vi "auto_Trans.vi"() -> ()   [LabVIEW 2016]
uses:
  <vilib>/Utility/miscctls.llb/LVOffsetAndMultiplierTypeDef.ctl
panel:
  in  "Tab Control":enum32{"Settings", "Raw", "Intensity"}(tab)
  out "Index":T1={"B Field"=1, "Voltage 2"=6, "Voltage 1"=4, "Current"=10, "Side Gate"=3, "Single/Differential 2"=FALSE} {"Side Gate" items=["time", "Vsg", "T", "B", "X0", "Y0", "X1", "Y1", "X2", "Y2", "X3", "Y3", "X4", "Y4", "X5", "Y5", "B_rate", "R4t(e2/h)", "axis1", "axis2", "20", "21", "22", "23", "24", "25", "26", "27", ""]; "Current" items=["time", "Vsg", "T", "B", "X0", "Y0", "X1", "Y1", "X2", "Y2", "X3", "Y3", "X4", "Y4", "X5", "Y5", "B_rate", "R4t(e2/h)", "axis1", "axis2", "20", "21", "22", "23", "24", "25", "26", "27", ""]; "Voltage 1" items=["time", "Vsg", "T", "B", "X0", "Y0", "X1", "Y1", "X2", "Y2", "X3", "Y3", "X4", "Y4", "X5", "Y5", "B_rate", "R4t(e2/h)", "axis1", "axis2", "20", "21", "22", "23", "24", "25", "26", "27", ""]; "Voltage 2" items=["time", "Vsg", "T", "B", "X0", "Y0", "X1", "Y1", "X2", "Y2", "X3", "Y3", "X4", "Y4", "X5", "Y5", "B_rate", "R4t(e2/h)", "axis1", "axis2", "20", "21", "22", "23", "24", "25", "26", "27", ""]; "B Field" items=["time", "Vsg", "T", "B", "X0", "Y0", "X1", "Y1", "X2", "Y2", "X3", "Y3", "X4", "Y4", "X5", "Y5", "B_rate", "R4t(e2/h)", "axis1", "axis2", "20", "21", "22", "23", "24", "25", "26", "27", ""]}
  in  "Derivative Bin \nSize":dbl=20.0
  out "Comments":string="IGOR\nX// Date: 1/22/2017 12:53 AM\nX// sweep B: 0T to 18T and 18T to 0T, @ 0.02 T/min\nX// sweep Vsg: 0mV to 120mV, 250uV steps\nX// Vbg=0.3V\nX// T~20mK\nX// \nX// lockin settings: \nX// tc=0.3s\nX// order=4\nX// prefilters OFF\nX// \nX// 0: 1, voltage\nX// 1: 2, current, 100uV AC 240uV DC, 13 Hz\nX// 2: 3, voltage\nX// 3: 4, voltage\nX// 4: 5, current\nX// 5: 7, voltage\nX//  \nX// KH gian=100x, shurt resistor=50kOhm\nX// \nX// angle=167.007000\n\n\n\n\n\n\n\n\n\n\n\n\n\n\n\n\n\n\n\n\n\n\n\n\n\n\n\n\n\n\n\n\n\n\n\n\n\n\n\n\n\n\nX \nX Display/R 'time.SA02836H.20170110.000534'\nX AppendToGraph 'Vsg.SA02836H.20170110.000534'\nX AppendToGraph 'T.SA02836H.20170110.000534'\nX AppendToGraph 'B.SA02836H.20170110.000534'\nX AppendToGraph 'X0.SA02836H.20170110.000534'\nX AppendToGraph 'Y0.SA02836H.20170110.000534'\nX AppendToGraph 'X1.SA02836H.20170110.000534'\nX AppendToGraph 'Y1.SA02836H.20170110.000534'\nX AppendToGraph 'X2.SA02836H.20170110.000534'\nX AppendToGraph 'Y2.SA02836H.20170110.000534'\nX AppendToGraph 'X3.SA02836H.20170110.000534'\nX AppendToGraph 'Y3.SA02836H.20170110.000534'\nX AppendToGraph 'X4.SA02836H.20170110.000534'\nX AppendToGraph 'Y4.SA02836H.20170110.000534'\nX AppendToGraph 'X5.SA02836H.20170110.000534'\nX AppendToGraph 'Y5.SA02836H.20170110.000534'\nX AppendToGraph 'B_rate.SA02836H.20170110.000534'\nX AppendToGraph 'R4t(e2/h).SA02836H.20170110.000534'\nX AppendToGraph 'axis1.SA02836H.20170110.000534'\nX AppendToGraph 'axis2.SA02836H.20170110.000534'\nX Label bottom \"x label\"\nX Label left \"y label\"\nX ModifyGraph rgb('time.SA02836H.20170110.000534')=(65280,0,0)\nX ModifyGraph rgb('Vsg.SA02836H.20170110.000534')=(65280,18432,0)\nX ModifyGraph rgb('T.SA02836H.20170110.000534')=(65280,35328,0)\nX ModifyGraph rgb('B.SA02836H.20170110.000534')=(65280,52224,0)\nX ModifyGraph rgb('X0.SA02836H.20170110.000534')=(60416,65280,0)\nX ModifyGraph rgb('Y0.SA02836H.20170110.000534')=(41984,65280,0)\nX ModifyGraph rgb('X1.SA02836H.20170110.000534')=(25088,65280,0)\nX ModifyGraph rgb('Y1.SA02836H.20170110.000534')=(8192,65280,0)\nX ModifyGraph rgb('X2.SA02836H.20170110.000534')=(0,65280,10240)\nX ModifyGraph rgb('Y2.SA02836H.20170110.000534')=(0,65280,28672)\nX ModifyGraph rgb('X3.SA02836H.20170110.000534')=(0,65280,45568)\nX ModifyGraph rgb('Y3.SA02836H.20170110.000534')=(0,65280,62464)\nX ModifyGraph rgb('X4.SA02836H.20170110.000534')=(0,50176,65280)\nX ModifyGraph rgb('Y4.SA02836H.20170110.000534')=(0,31744,65280)\nX ModifyGraph rgb('X5.SA02836H.20170110.000534')=(0,14848,65280)\nX ModifyGraph rgb('Y5.SA02836H.20170110.000534')=(2048,0,65280)\nX ModifyGraph rgb('B_rate.SA02836H.20170110.000534')=(20480,0,65280)\nX ModifyGraph rgb('R4t(e2/h).SA02836H.20170110.000534')=(38912,0,65280)\nX ModifyGraph rgb('axis1.SA02836H.20170110.000534')=(55808,0,65280)\nX ModifyGraph rgb('axis2.SA02836H.20170110.000534')=(65280,0,58368)\nX Legend/C/N=text0/J \"\\\\s('time.SA02836H.20170110.000534') time\\r\\\\s('Vsg.SA02836H.20170110.000534') Vsg\\r\\\\s('T.SA02836H.20170110.000534') T\\r\\\\s('B.SA02836H.20170110.000534') B\\r\\\\s('X0.SA02836H.20170110.000534') X0\\r\\\\s('Y0.SA02836H.20170110.000534') Y0\\r\\\\s('X1.SA02836H.20170110.000534') X1\\r\\\\s('Y1.SA02836H.20170110.000534') Y1\\r\\\\s('X2.SA02836H.20170110.000534') X2\\r\\\\s('Y2.SA02836H.20170110.000534') Y2\\r\\\\s('X3.SA02836H.20170110.000534') X3\\r\\\\s('Y3.SA02836H.20170110.000534') Y3\\r\\\\s('X4.SA02836H.20170110.000534') X4\\r\\\\s('Y4.SA02836H.20170110.000534') Y4\\r\\\\s('X5.SA02836H.20170110.000534') X5\\r\\\\s('Y5.SA02836H.20170110.000534') Y5\\r\\\\s('B_rate.SA02836H.20170110.000534') B_rate\\r\\\\s('R4t(e2/h).SA02836H.20170110.000534') R4t (e2/h)\\r\\\\s('axis1.SA02836H.20170110.000534') axis 1\\r\\\\s('axis2.SA02836H.20170110.000534') axis 2\"\nX ModifyGraph mirror(bottom)=1\nX ModifyGraph width=216\nX ModifyGraph height={Aspect,0.6}\nX ModifyGraph Log(bottom)=0\nX ModifyGraph Log(left)=0\nX \n"
  in  "Index":bool
  in  "Path":path=path "C:/LevyLab/LevyLab Projects/automation/files"
  in  "Index.":T2={"Side Gate"=1, "Current"=12, "Voltage 1"=8, "Voltage 2"=10, "B Field"=3, "Single/Differential 2"=TRUE}
  in  "Stop":bool
  out "Transconductance":T3(graph)
  out "Conductance":T3(graph)
  out "String 2":string="Transconductance"
  out "String":string="Conductance"
  out "Transconductance..":dbl[][](graph)
  out "String 4":string="Transconductance"
  out "Conductance..":dbl[][](graph)
  out "String 3":string="Conductance"
  out "Added?":string="Handle Closed"
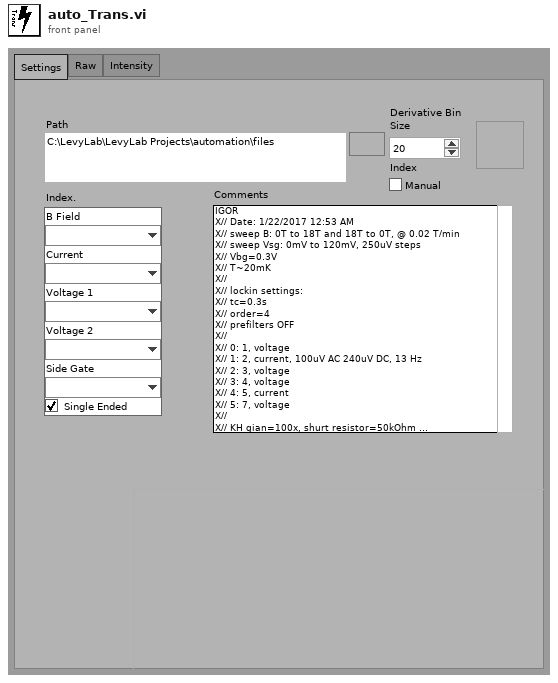
[diagram p1: front panel]
types:
  T1 = cluster{"B Field":i32, "Voltage 2":i32, "Voltage 1":i32, "Current":i32, "Side Gate":i32, "Single/Differential 2":bool}
  T2 = cluster{"Side Gate":i32, "Current":i32, "Voltage 1":i32, "Voltage 2":i32, "B Field":i32, "Single/Differential 2":bool}
  T3 = cluster{"Vfast":dbl[], "Decimated Array":dbl[]}[]
  T4 = enum32{"invalid app kind", "Development System", "Run Time System", "Student Edition", "Embedded LabVIEW", "Evaluation", "Custom"}
  T5 = enum32{"Invalid", "Standard", "Closed", "Hidden", "Minimized", "Maximized"}
  T6 = typedef "LVOffsetAndMultiplierTypeDef.ctl" = cluster{"Offset":dbl, "Multiplier":dbl}
  T7 = cluster{"N1":i32, "N2":i32, "N3":i32, "N4":i32, "V1":i32, "V2":i32, "V3":i32, "V4":i32, "CURRENT":i32, "Vsg":i32}
  T8 = cluster{"Core":cluster{"Current VI Reference":refnum<vi>, "Close Panel on Exit?":bool}, "Boolean Values":cluster{"Your Boolean data":bool, "single ended?":bool}, "Your string data":string, "Paths":cluster{"Path":path}, "Graphs":cluster{"Cond.":cluster{dbl[], dbl[]}[], "Trans.":cluster{"Vfast":dbl[], "Decimated Array":dbl[]}[], "Cond. Intens.":dbl[][], "Trans. Intens.":dbl[][], "Cond. Intens. bg":dbl[][], "Trans. Intens. bg":dbl[][]}, "Index/ Comments":cluster{"Comments":string, "Index":cluster{"N1":i32, "N2":i32, "N3":i32, "N4":i32, "V1":i32, "V2":i32, "V3":i32, "V4":i32, "CURRENT":i32, "Vsg":i32}, "Wavenames":string[]}, "Images":cluster{"Image":picture}, "B Field":i32}
  T9 = cluster{"Comments":string, "Index":cluster{"N1":i32, "N2":i32, "N3":i32, "N4":i32, "V1":i32, "V2":i32, "V3":i32, "V4":i32, "CURRENT":i32, "Vsg":i32}, "Wavenames":string[]}
  T10 = cluster{"Your Boolean data":bool, "single ended?":bool}
  T11 = cluster{"Cond.":cluster{dbl[], dbl[]}[], "Trans.":cluster{"Vfast":dbl[], "Decimated Array":dbl[]}[], "Cond. Intens.":dbl[][], "Trans. Intens.":dbl[][], "Cond. Intens. bg":dbl[][], "Trans. Intens. bg":dbl[][]}
  T12 = cluster{"Current VI Reference":refnum<vi>, "Close Panel on Exit?":bool}
  T13 = cluster{"Side Gate":i32, "Current":i32, "Voltage 1":i32, "Voltage 2":i32, "B Field":i32, "Voltage":bool}
  T14 = cluster{"Decimated Array":dbl[], "Decimated Array":dbl[]}
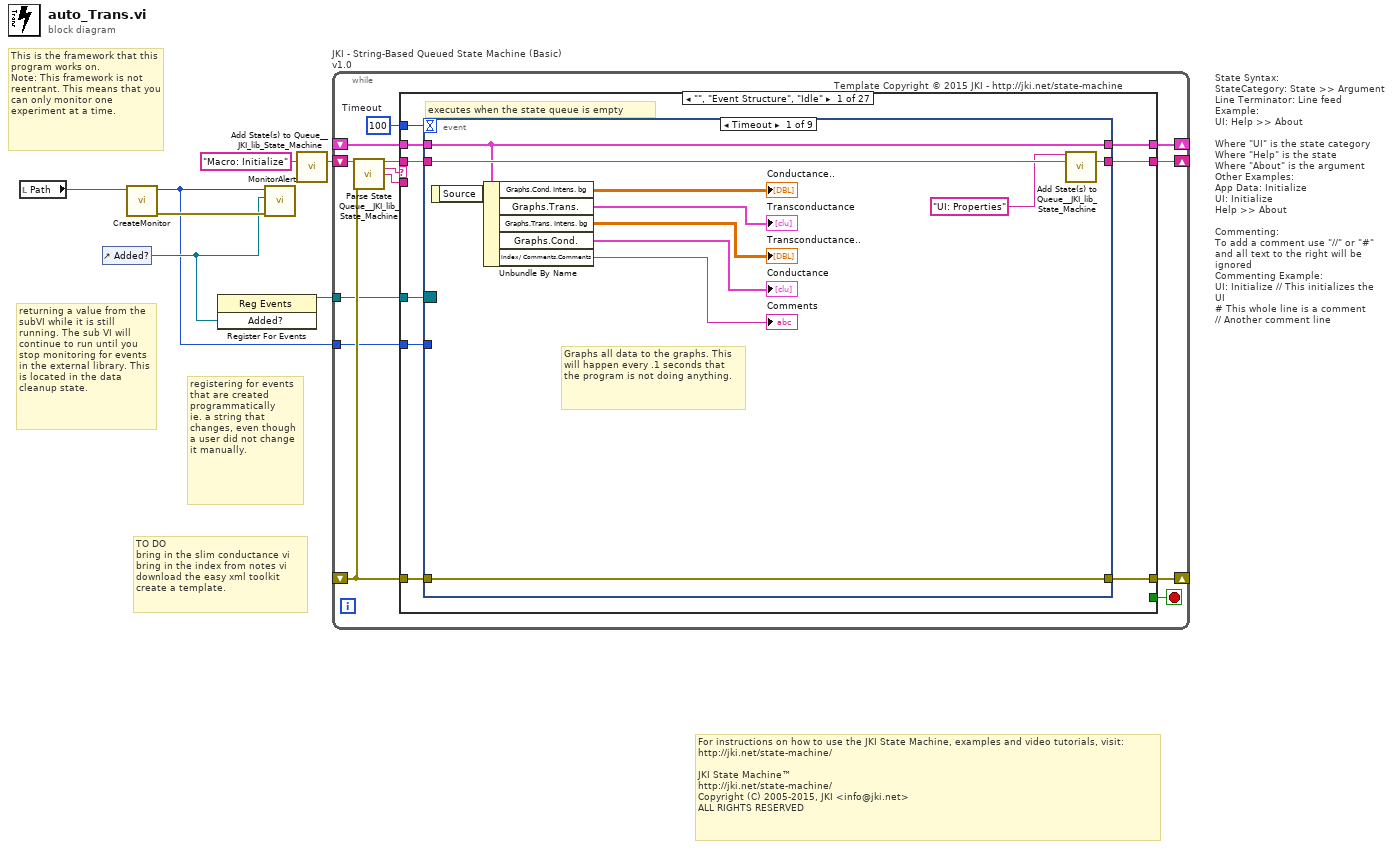
[diagram p0: block diagram]
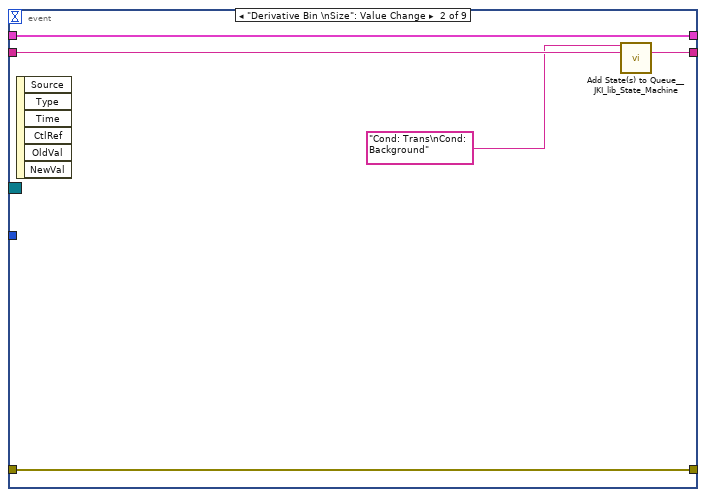
[diagram p2: hidden frame]
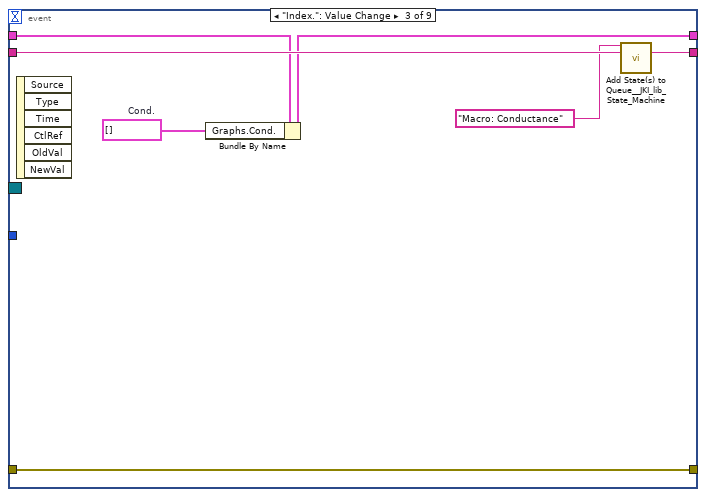
[diagram p3: hidden frame]
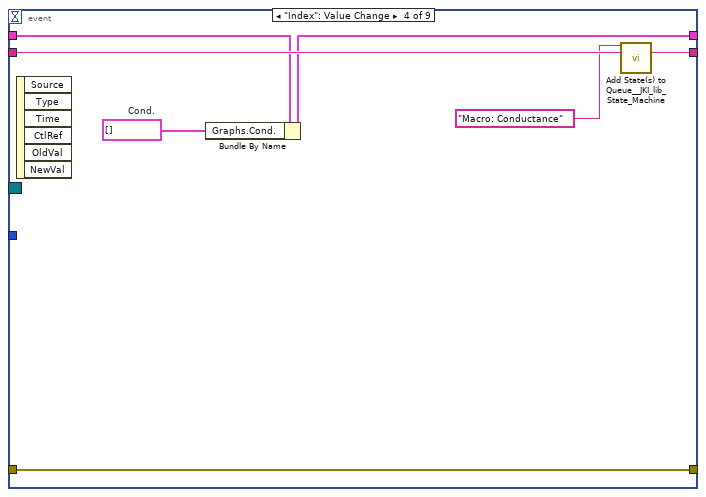
[diagram p4: hidden frame]
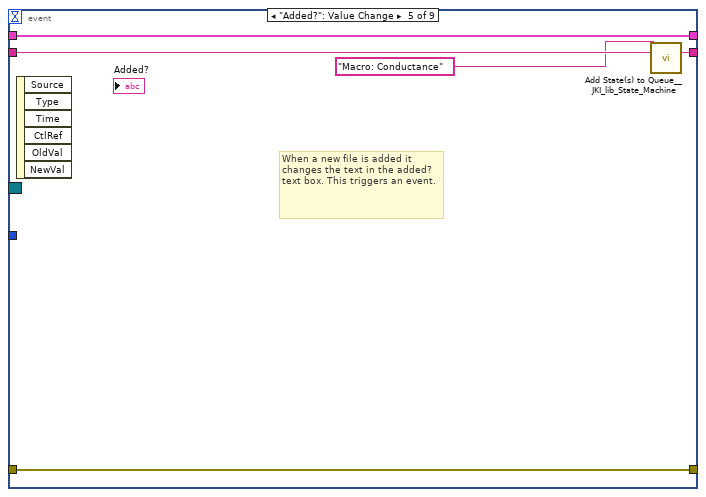
[diagram p5: hidden frame]
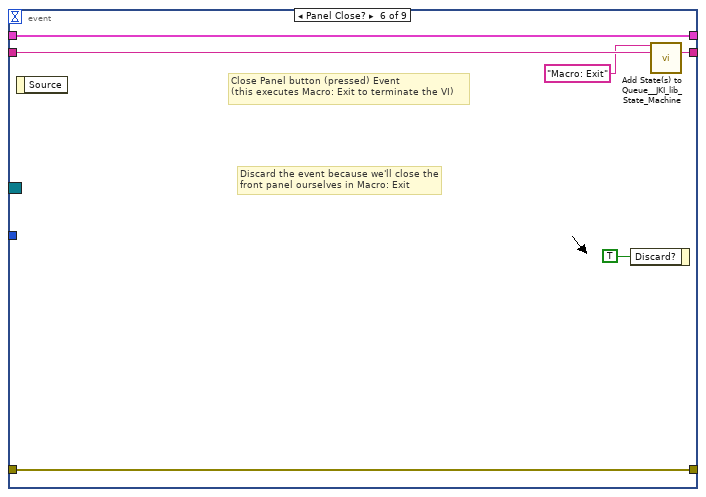
[diagram p6: hidden frame]
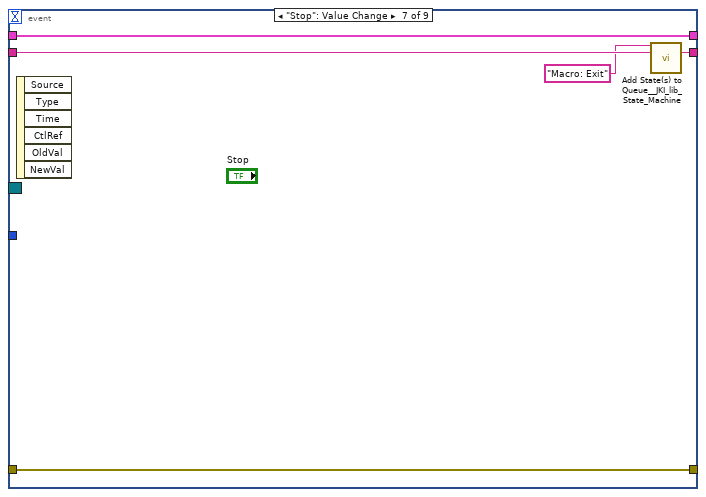
[diagram p7: hidden frame]
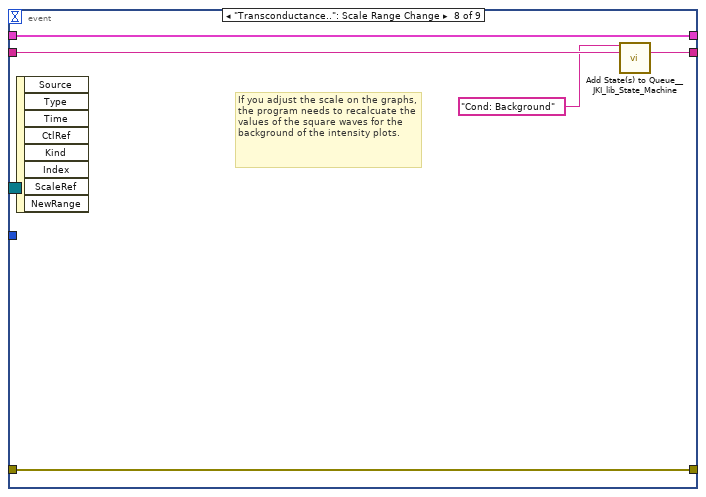
[diagram p8: hidden frame]
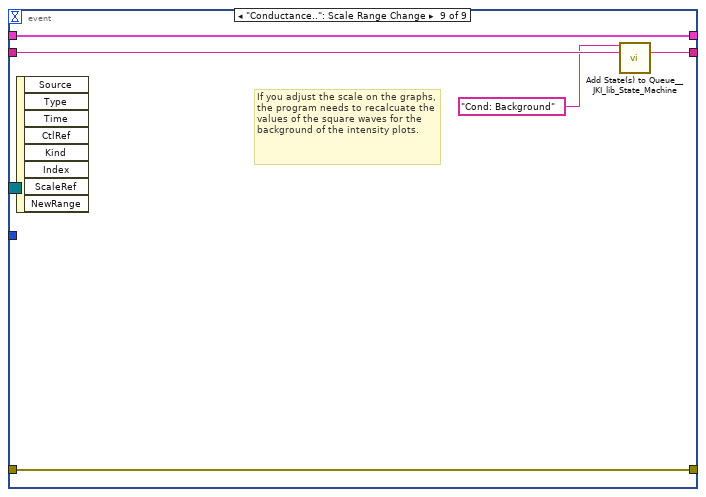
[diagram p9: hidden frame]
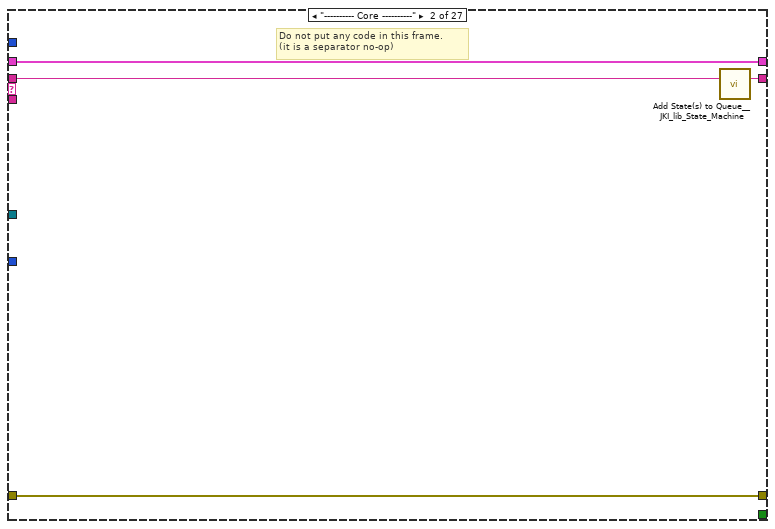
[diagram p10: hidden frame]
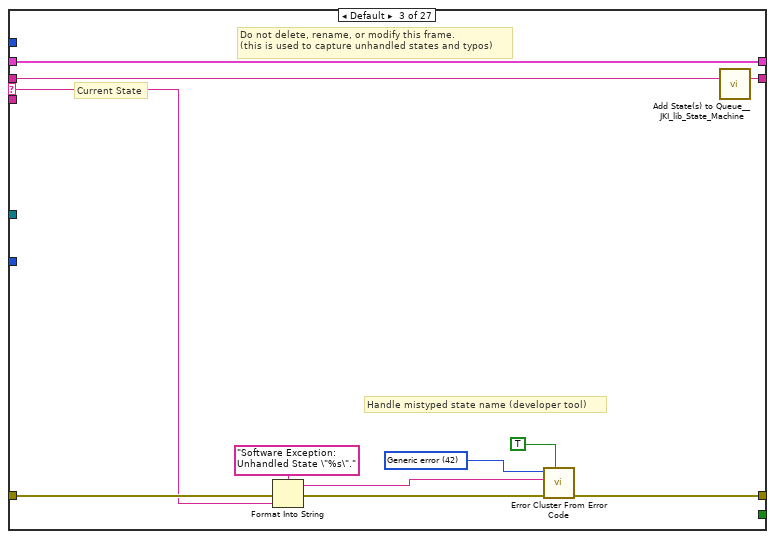
[diagram p11: hidden frame]
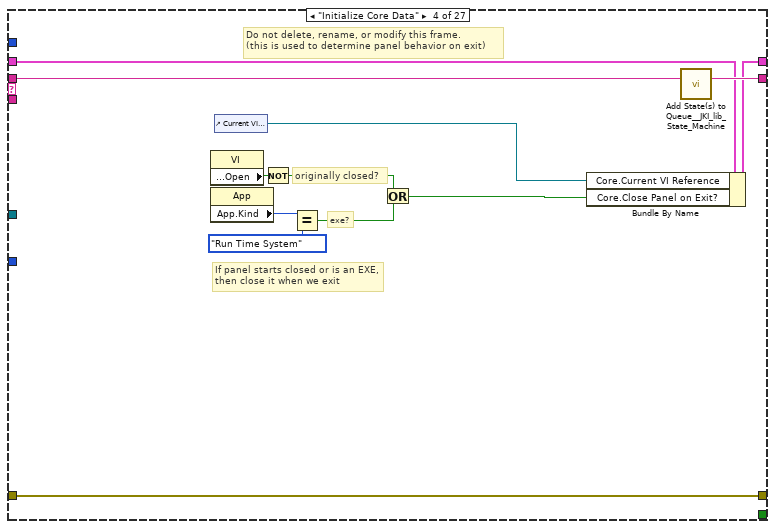
[diagram p12: hidden frame]
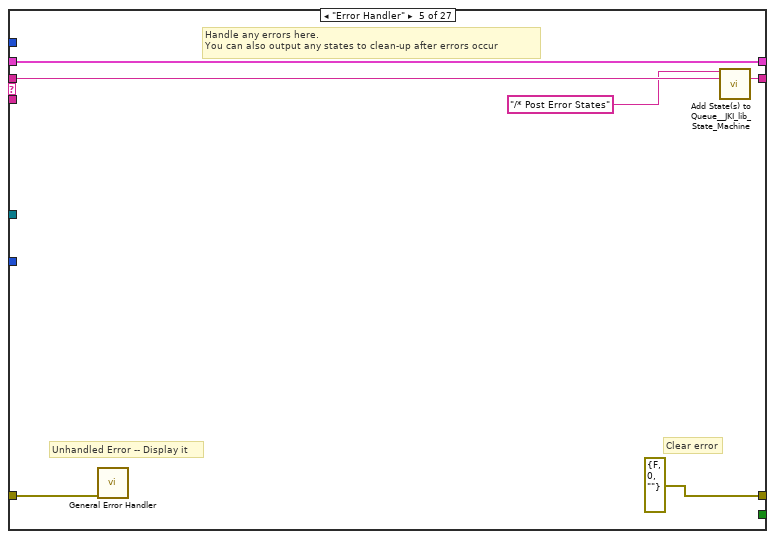
[diagram p13: hidden frame]
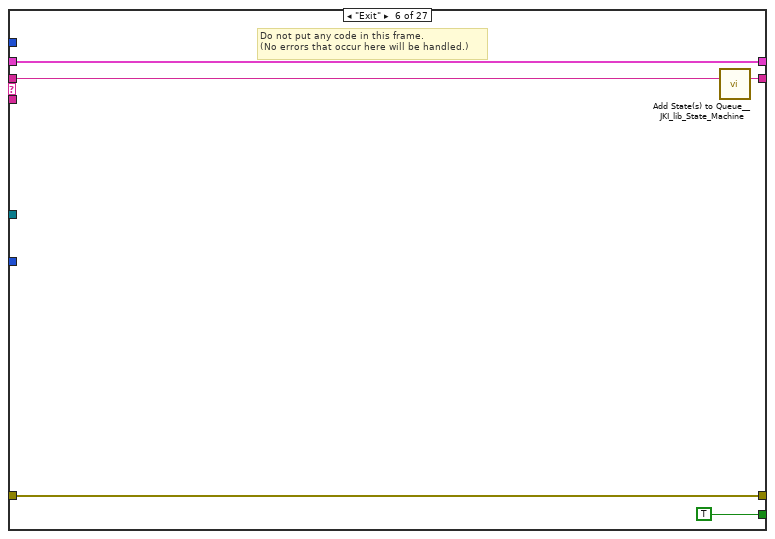
[diagram p14: hidden frame]
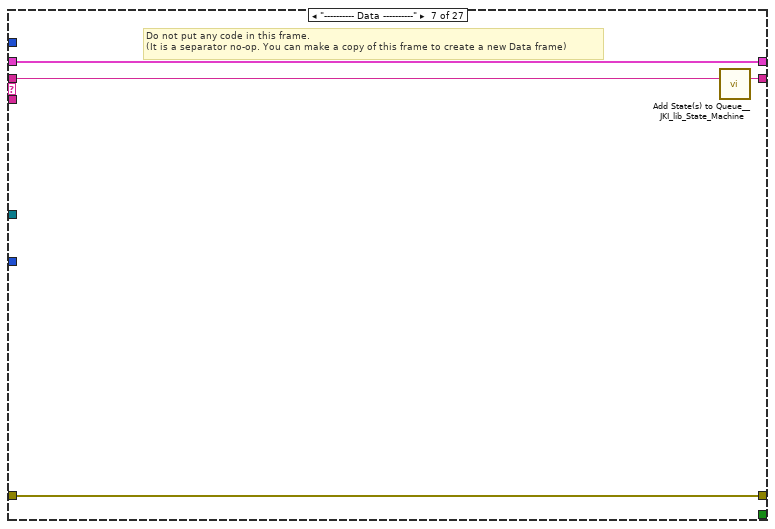
[diagram p15: hidden frame]
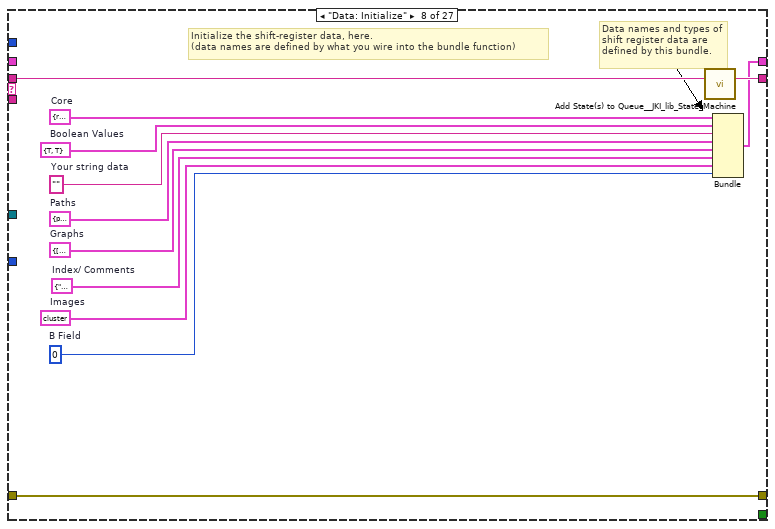
[diagram p16: hidden frame]
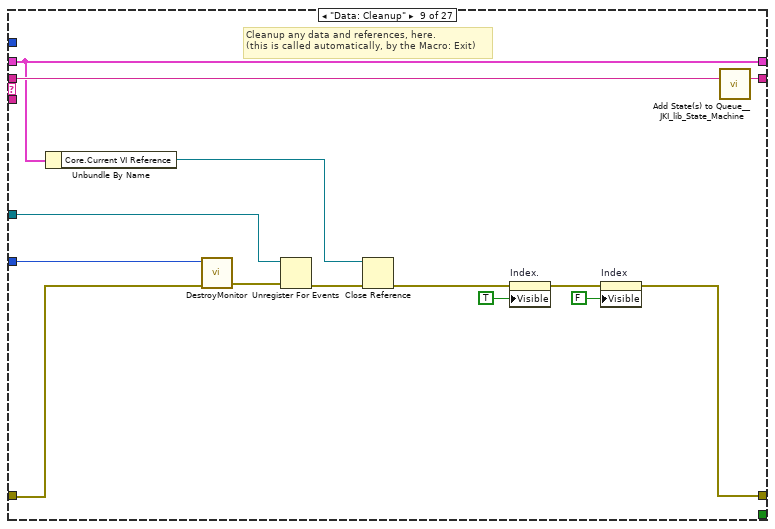
[diagram p17: hidden frame]
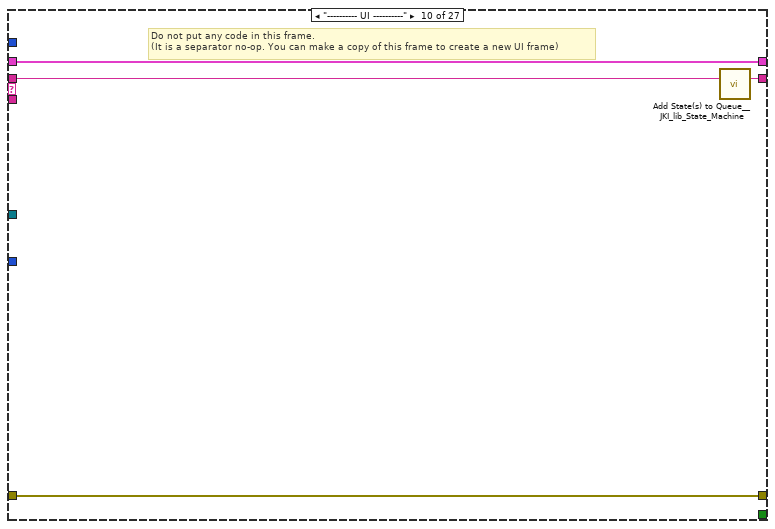
[diagram p18: hidden frame]
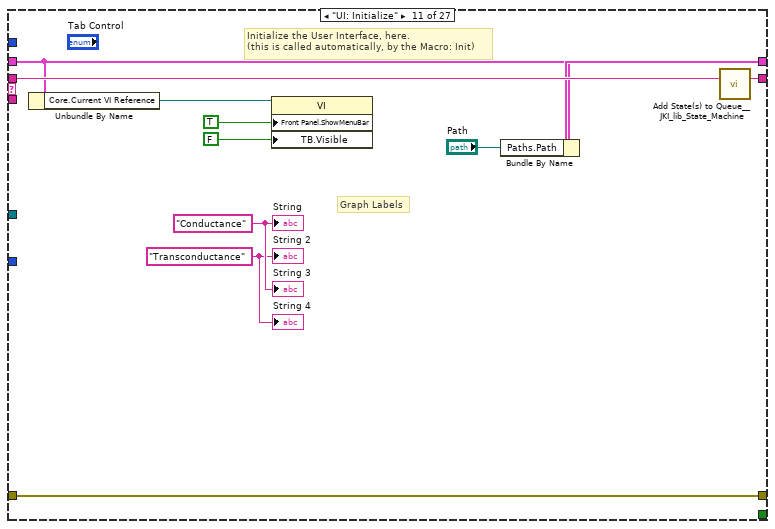
[diagram p19: hidden frame]
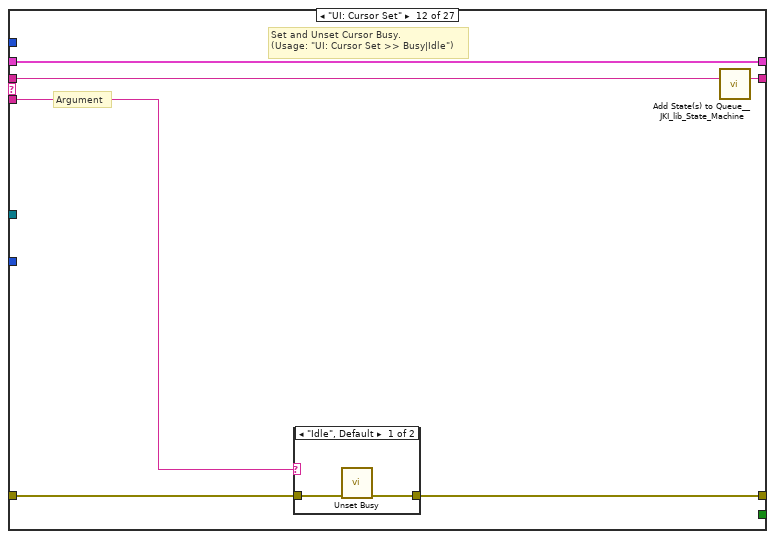
[diagram p20: hidden frame]
diagram:
  # "TO DO\nbring in the slim conductance vi\nbring in the index from notes vi\ndownload the easy xml toolkit\ncreate a template."
  # "registering for events that are created programmatically\nie. a string that changes, even though a user did not change it manually."
  # "returning a value from the subVI while it is still running. The sub VI will continue to run until you stop monitoring for events in the external library. This is located in the data cleanup state."
  # "This is the framework that this program works on.\nNote: This framework is not reentrant. This means that you can only monitor one experiment at a time."
  # "State Syntax:\nStateCategory: State >> Argument\nLine Terminator: Line feed\nExample:\nUI: Help >> About\n\nWhere \"UI\" is the state category\nWhere \"Help\" is the state\nWhere \"About\" is the argument\nOther Examples:\nApp Data: Initialize\nUI: Initialize\nHelp >> About\n\nCommenting:\nTo add a comment use \"//\" or \"#\" and all text to the right will be ignored\nCommenting Example:\nUI: Initialize // This initializes the UI\n# This whole line is a comment\n// Another comment line"
  # "For instructions on how to use the JKI State Machine, examples and video tutorials, visit:\nhttp://jki.net/state-machine/\n\nJKI State Machine™\nhttp://jki.net/state-machine/\nCopyright (C) 2005-2015, JKI <info@jki.net>\nALL RIGHTS RESERVED"
  n1 = local read "Path"() -> (w1:path)
  n2 = control-ref of="Added?"() -> (w4:refnum<vi>)
  n3 = call "CreateMonitor.vi"("File Path Control"=w1) -> ("error out"=w5:errorcluster, "Handle"=w2:i32)  [unwired: 9 in]
  n4 = register-events(w4) -> (reference out=w3:refnum<event-registration>)  [unwired: 2 in, 1 out]
  n5 = call "MonitorAlert.vi"("error in (no error)"=w5, "Str Refnum"=w4, "Handle"=w2) -> ()  [unwired: 8 in, 1 out]
  n6 = call <vilib>:"Add State(s) to Queue__JKI_lib_State_Machine.vi"("State(s) in (\"\")"="Macro: Initialize") -> ("States Out"=w7:string)  [unwired: 14 in]
  n7 = while "JKI - String-Based Queued State Machine (Basic) v1.0" {
    shift-right: [w13] -> _
    shift-left: _ -> [w12]
    shift-right: [w16] -> _
    shift-left: _ -> [w10]
    shift-right: [w15] -> _
    shift-left: w7 -> [w17]
    tunnel: w3 -> [w9]
    tunnel: w2 -> [w8]
    stop <- w14 stop-if-true
    w11 = 100  # Timeout
    # "Template Copyright © 2015 JKI - http://jki.net/state-machine"
    n8 = call <vilib>:"Parse State Queue__JKI_lib_State_Machine.vi"("State Queue"=w17, "Error In (no error)"=w10) -> ("Remaining States"=w19:string, "Current State"=w20:string, "Arguments"=w18:string)  [unwired: 11 in]
    n9 = case shown="\"\", \"Event Structure\", \"Idle\"" w20 {
      selector: w20 -> [_ _ w89 _ _ _ _ _ _ _ _ _ _ _ _ _ _ _ _ _ _ _ _ _ _ _ _]
      tunnel: w19 -> [w29 w88 w93 w111 w117 w122 w126 w138 w152 w156 w167 w173 w184 w228 w234 w239 w244 w254 w258 w269 w273 w294 w315 w325 w343 w347 w351]
      tunnel: w18 -> [_ _ _ _ _ _ _ _ _ _ _ w168 w178 _ _ _ _ _ _ _ _ _ _ _ _ _ _]
      tunnel: w12 -> [w27 w85 w91 w102 w114 w120 w123 _ w150 w153 w163 w171 w180 w225 w231 w236 w241 w252 w255 w267 w270 w287 w311 w318 w340 w344 w348]
      tunnel: [w26 w86 w95 w108 errorcluster {"status"=FALSE, "code"=0, "source"=""} ("error out") w119 w124 w135 w140 w154 w164 w169 w181 w226 w232 w237 w242 w245 w256 w259 w271 w292 w313 w323 w341 w345 w349] -> w16
      tunnel: w10 -> [w25 w86 w94 w108 w113 w119 w124 w135 w144 w154 w164 w170 w182 w226 w232 w237 w242 w245 w256 w260 w271 w292 w313 w323 w341 w345 w349]
      tunnel: [w28 w87 w92 w110 w116 w121 w125 w137 w151 w155 w166 w172 w183 w227 w233 w238 w243 w253 w257 w268 w272 w293 w314 w324 w342 w346 w350] -> w15
      tunnel: [_ _ _ _ _ TRUE _ _ _ _ _ _ _ _ _ _ _ _ _ _ _ _ _ _ _ _ _] -> w14
      tunnel: [w24 w85 w91 w109 w114 w120 w123 w136 w150 w153 w165 w171 w180 w225 w231 w236 w241 w252 w255 w267 w270 w286 w312 w320 w339 w344 w348] -> w13
      tunnel: w11 -> [w23 _ _ _ _ _ _ _ _ _ _ _ _ _ _ _ _ _ _ _ _ _ _ _ _ _ _]
      tunnel: w9 -> [w22 _ _ _ _ _ _ _ w148 _ _ _ _ _ _ _ _ _ _ _ _ _ _ _ _ _ _]
      tunnel: w8 -> [w21 _ _ _ _ _ _ _ w149 _ _ _ _ _ _ _ _ _ _ _ _ _ _ _ _ _ _]
      frame "", "Event Structure", "Idle" {
        # "executes when the state queue is empty"
        n10 = event shown="[0] Timeout" {
          selector: w22 -> [_ _ _ _ _ _ _ _ _]
          dyn-events: _ -> [_ _ _ _ _ _ _ _ _]
          timeout: w23 -> [_ _ _ _ _ _ _ _ _]
          tunnel: w29 -> [w39 w42 w49 w56 w63 w69 w74 w77 w82]
          tunnel: [w38 w43 w50 w57 w62 w68 w73 w78 w83] -> w28
          tunnel: w27 -> [w36 w41 w46 w53 w61 w66 w71 w79 w84]
          tunnel: [w37 w44 w51 w58 w60 w67 w72 w75 w80] -> w26
          tunnel: w25 -> [w37 w44 w51 w58 w60 w67 w72 w75 w80]
          tunnel: [w36 w41 w45 w52 w61 w66 w71 w79 w84] -> w24
          tunnel: w21 -> [_ _ _ _ _ _ _ _ _]
          event Timeout {
            # "Graphs all data to the graphs. This will happen every .1 seconds that the program is not doing anything."
            n11 = event-data() -> ()  [unwired: 1 in, 1 out]
            n12 = Unbundle By Name(w36) -> ("Graphs.Cond. Intens. bg"=→"Conductance..":dbl[][], "Graphs.Trans."=→"Transconductance":T3, "Graphs.Trans. Intens. bg"=→"Transconductance..":dbl[][], "Graphs.Cond."=→"Conductance":cluster{dbl[], dbl[]}[], "Index/ Comments.Comments"=→"Comments":string)
            n13 = call <vilib>:"Add State(s) to Queue__JKI_lib_State_Machine.vi"("State(s) in Front (\"\")"="UI: Properties" ("State(s) in Front (\"\")"), "State(s) in (\"\")"=w39) -> ("States Out"=w38:string)  [unwired: 13 in]
          }
          event "Derivative Bin \nSize": Value Change {
            n14 = event-data() -> ()  [unwired: 1 in, 6 out]
            n15 = call <vilib>:"Add State(s) to Queue__JKI_lib_State_Machine.vi"("State(s) in Front (\"\")"="Cond: Trans\nCond: Background" ("State(s) in Front (\"\")"), "State(s) in (\"\")"=w42) -> ("States Out"=w43:string)  [unwired: 13 in]
          }
          event "Index.": Value Change {
            w48 = cluster{dbl[], dbl[]}[] []  # Cond.
            n16 = event-data() -> ()  [unwired: 1 in, 6 out]
            n17 = Bundle By Name(cluster=w46, "Graphs.Cond."=w48) -> (w45:T8)
            n18 = call <vilib>:"Add State(s) to Queue__JKI_lib_State_Machine.vi"("State(s) in Front (\"\")"="Macro: Conductance" ("State(s) in Front (\"\")"), "State(s) in (\"\")"=w49) -> ("States Out"=w50:string)  [unwired: 13 in]
          }
          event "Index": Value Change {
            w55 = cluster{dbl[], dbl[]}[] []  # Cond.
            n19 = event-data() -> ()  [unwired: 1 in, 6 out]
            n20 = Bundle By Name(cluster=w53, "Graphs.Cond."=w55) -> (w52:T8)
            n21 = call <vilib>:"Add State(s) to Queue__JKI_lib_State_Machine.vi"("State(s) in Front (\"\")"="Macro: Conductance" ("State(s) in Front (\"\")"), "State(s) in (\"\")"=w56) -> ("States Out"=w57:string)  [unwired: 13 in]
          }
          event "Added?": Value Change {
            # "When a new file is added it changes the text in the added? text box. This triggers an event."
            n22 = event-data() -> ()  [unwired: 1 in, 6 out]
            n23 = call <vilib>:"Add State(s) to Queue__JKI_lib_State_Machine.vi"("State(s) in Front (\"\")"="Macro: Conductance" ("State(s) in Front (\"\")"), "State(s) in (\"\")"=w63) -> ("States Out"=w62:string)  [unwired: 13 in]
          }
          event Panel Close? {
            # "Discard the event because we'll close the front panel ourselves in Macro: Exit"
            # "Close Panel button (pressed) Event\n(this executes Macro: Exit to terminate the VI)"
            n24 = event-data() -> ()  [unwired: 1 in, 1 out]
            n25 = event-data("Discard?"=TRUE) -> ()  [unwired: 1 in, 1 out]
            n26 = call <vilib>:"Add State(s) to Queue__JKI_lib_State_Machine.vi"("State(s) in Front (\"\")"="Macro: Exit", "State(s) in (\"\")"=w69) -> ("States Out"=w68:string)  [unwired: 13 in]
          }
          event "Stop": Value Change {
            n27 = event-data() -> ()  [unwired: 1 in, 6 out]
            n28 = call <vilib>:"Add State(s) to Queue__JKI_lib_State_Machine.vi"("State(s) in Front (\"\")"="Macro: Exit", "State(s) in (\"\")"=w74) -> ("States Out"=w73:string)  [unwired: 13 in]
          }
          event "Transconductance..": Scale Range Change {
            # "If you adjust the scale on the graphs, the program needs to recalcuate the values of the square waves for the background of the intensity plots."
            n29 = event-data() -> ()  [unwired: 1 in, 8 out]
            n30 = call <vilib>:"Add State(s) to Queue__JKI_lib_State_Machine.vi"("State(s) in Front (\"\")"="Cond: Background" ("State(s) in Front (\"\")"), "State(s) in (\"\")"=w77) -> ("States Out"=w78:string)  [unwired: 13 in]
          }
          event "Conductance..": Scale Range Change {
            # "If you adjust the scale on the graphs, the program needs to recalcuate the values of the square waves for the background of the intensity plots."
            n31 = event-data() -> ()  [unwired: 1 in, 8 out]
            n32 = call <vilib>:"Add State(s) to Queue__JKI_lib_State_Machine.vi"("State(s) in Front (\"\")"="Cond: Background" ("State(s) in Front (\"\")"), "State(s) in (\"\")"=w82) -> ("States Out"=w83:string)  [unwired: 13 in]
          }
        }
      }
      frame "---------- Core ----------" {
        # "Do not put any code in this frame.\n(it is a separator no-op)"
        n33 = call <vilib>:"Add State(s) to Queue__JKI_lib_State_Machine.vi"("State(s) in (\"\")"=w88) -> ("States Out"=w87:string)  [unwired: 14 in]
      }
      frame Default {
        w98 = 42 items=["No error", "Argument error", "Memory is full", "Out of zone", "End of file", "File already open", "Generic file I/O error", "File not found", "File permission error", "Disk is full", "Duplicate path", "Too many files open", "System feature not enabled", "Resource file not found", "Cannot add resource", "Resource not found", "Image not found", "Image memory error", "Pen does not exist", "Config type invalid", "Config token not found", "Config parse error", "Config memory error", "Bad external code format", "Bad external code offset", "External code not present", "Null window", "Destroy window error", "Null menu", "Print aborted", "Bad print record", "Print driver error", "Windows error during printing", "Memory error during printing", "Print dialog error", "Generic print error", "Invalid device refnum", "Device not found", "Device parameter error", "Device unit error", "Cannot open device", "Device call aborted", "Generic error", "Cancelled by user", "Object ID too low", "Object ID too high", "Object not in heap", "Unknown heap", "Unknown object (invalid DefProc)", "Unknown object (DefProc not in table)", "Message out of range", "Invalid (null) method", "Unknown message", "Manager call not supported", "Bad address", "Network operation in progress", "Network operation timed out", "Connection is busy", "Network attribute not supported", "Network error", "Address in use", "System out of memory", "Connection aborted", "Connection refused", "Not connected", "Already connected", "Connection closed", "Initialization error (interapplication manager)", "Bad occurrence", "Wait on unbound occurrence handler", "Occurrence queue overflow", "Datalog type conflict", "Unused", "Unrecognized type (interapplication manager)", "Memory corrupt", "Failed to make temporary DLL", "Old CIN version", "Drag socket not found", "Failed to load drop-object", "Failed to register OLE object", "Failed to release OLE object", "Format specifier type mismatch", "Unknown format specifier", "Too few format specifiers", "Too many format specifiers", "Scan failed", "Newer CIN version", "Error converting to variant", "Runtime menu error", "Password tampered", "Variant attribute not found", "Incompatible variant data type", "Event data is not available", "Event Store is not present", "Occurrence is not found", "Event Queue is not created", "Event info is not available", "Refnum passed is NULL", "Error retrieving Class GUID", "Error retrieving CoClass GUID", "Error retrieving TypeLib GUID.", "Bad built application magic bytes.", "Specific driver is different from the specific driver associated with the Logical Name.", "There is no session opened to the class driver.", "Max Error", "MAX - Error with config objects", "MAX - Error loading configuration", "MAX - Group not supported"]
        # "Current State"
        # "Do not delete, rename, or modify this frame.\n(this is used to capture unhandled states and typos)"
        # "Handle mistyped state name (developer tool)"
        n34 = Format Into String(format string="Software Exception: Unhandled State \"%s\"." ("message"), error in=w94, w89) -> (resulting string=w97:string, error out=w96:errorcluster)  [unwired: 1 in]
        n35 = call <vilib>:"Error Cluster From Error Code.vi"("show call chain? (False)"=TRUE, "error in (no error)"=w96, "error message (\"\")"=w97, "error code (0)"=w98) -> ("error out"=w95:errorcluster)  [unwired: 5 in]
        n36 = call <vilib>:"Add State(s) to Queue__JKI_lib_State_Machine.vi"("State(s) in (\"\")"=w93) -> ("States Out"=w92:string)  [unwired: 14 in]
      }
      frame "Initialize Core Data" {
        # "Do not delete, rename, or modify this frame.\n(this is used to determine panel behavior on exit)"
        # "originally closed?"
        # "exe?"
        # "If panel starts closed or is an EXE, then close it when we exit"
        n37 = property class="VI"() -> ("Front Panel.Open"=w107:bool)  [unwired: 2 in, 2 out]
        n38 = property class="App"() -> ("App.Kind"=w106:T4)  [unwired: 2 in, 2 out]
        n39 = control-ref of="Current VI Reference"() -> (w100:refnum<vi>)
        n40 = Not(x=w107) -> (.not. x?=w104:bool)
        n41 = Equal?(x=w106, y=T4."Run Time System" ("Application:Kind")) -> (x = y?=w103:bool)
        n42 = Or(x=w104, y=w103) -> (x .or. y?=w101:bool)
        n43 = Bundle By Name(cluster=w102, "Core.Current VI Reference"=w100, "Core.Close Panel on Exit?"=w101) -> (w109:T8)
        n44 = call <vilib>:"Add State(s) to Queue__JKI_lib_State_Machine.vi"("State(s) in (\"\")"=w111) -> ("States Out"=w110:string)  [unwired: 14 in]
      }
      frame "Error Handler" {
        # "Unhandled Error -- Display it"
        # "Handle any errors here.\nYou can also output any states to clean-up after errors occur"
        # "Clear error"
        n45 = call <vilib>:"General Error Handler.vi"("error in (no error)"=w113) -> ()  [unwired: 10 in, 5 out]
        n46 = call <vilib>:"Add State(s) to Queue__JKI_lib_State_Machine.vi"("State(s) in Front (\"\")"="/* Post Error States", "State(s) in (\"\")"=w117) -> ("States Out"=w116:string)  [unwired: 13 in]
      }
      frame "Exit" {
        # "Do not put any code in this frame.\n(No errors that occur here will be handled.)"
        n47 = call <vilib>:"Add State(s) to Queue__JKI_lib_State_Machine.vi"("State(s) in (\"\")"=w122) -> ("States Out"=w121:string)  [unwired: 14 in]
      }
      frame "---------- Data ----------" {
        # "Do not put any code in this frame.\n(It is a separator no-op. You can make a copy of this frame to create a new Data frame)"
        n48 = call <vilib>:"Add State(s) to Queue__JKI_lib_State_Machine.vi"("State(s) in (\"\")"=w126) -> ("States Out"=w125:string)  [unwired: 14 in]
      }
      frame "Data: Initialize" {
        w127 = 0  # B Field
        w128 = cluster{"Image":picture} {"Image"=bytes[0]}  # Images
        w129 = cluster{"Path":path} {"Path"=path ""}  # Paths
        w130 = T9 {"Comments"="", "Index"={"N1"=0, "N2"=0, "N3"=0, "N4"=0, "V1"=0, "V2"=0, "V3"=0, "V4"=0, "CURRENT"=0, "Vsg"=0}, "Wavenames"=["time", "Vsg", "T", "B", "X0", "Y0", "X1", "Y1", "X2", "Y2", "X3", "Y3", "X4", "Y4", "X5", "Y5", "B_rate", "R4t(e2/h)", "axis1", "axis2", ""]}  # Index/ Comments
        w131 = T10 {"Your Boolean data"=TRUE, "single ended?"=TRUE}  # Boolean Values
        w132 = T11 {"Cond."=[], "Trans."=[], "Cond. Intens."=[], "Trans. Intens."=[], "Cond. Intens. bg"=[], "Trans. Intens. bg"=[]}  # Graphs
        w133 = T12 {"Current VI Reference"=refnum, "Close Panel on Exit?"=FALSE}  # Core
        w134 = ""  # Your string data
        # "Data names and types of shift register data are defined by this bundle."
        # "Initialize the shift-register data, here.\n(data names are defined by what you wire into the bundle function)"
        n49 = call <vilib>:"Add State(s) to Queue__JKI_lib_State_Machine.vi"("State(s) in (\"\")"=w138) -> ("States Out"=w137:string)  [unwired: 14 in]
        n50 = Bundle("Core"=w133, "Boolean Values"=w131, "Your string data"=w134, "Paths"=w129, "Graphs"=w132, "Index/ Comments"=w130, "Images"=w128, "B Field"=w127) -> (w136:T8)  [unwired: 1 in]
      }
      frame "Data: Cleanup" {
        # "Cleanup any data and references, here.\n(this is called automatically, by the Macro: Exit)"
        n51 = Unbundle By Name(w150) -> ("Core.Current VI Reference"=w145:refnum<vi>)
        n52 = call "DestroyMonitor.vi"("Error In"=w144, "Handle in"=w149) -> ("Error Out"=w147:errorcluster)  [unwired: 9 in]
        n53 = Unregister For Events(event registration refnum=w148, error in=w147) -> (error out=w146:errorcluster)
        n54 = Close Reference(reference=w145, error in (no error)=w146) -> (error out=w142:errorcluster)
        n55 = property on="Index." class="Clust (strict)"(error in=w142, "Visible"=TRUE) -> (error out=w141:errorcluster)  [unwired: 1 in, 1 out]
        n56 = property on="Index" class="Clust (strict)"(error in=w141, "Visible"=FALSE) -> (error out=w140:errorcluster)  [unwired: 1 in, 1 out]
        n57 = call <vilib>:"Add State(s) to Queue__JKI_lib_State_Machine.vi"("State(s) in (\"\")"=w152) -> ("States Out"=w151:string)  [unwired: 14 in]
      }
      frame "---------- UI ----------" {
        # "Do not put any code in this frame.\n(It is a separator no-op. You can make a copy of this frame to create a new UI frame)"
        n58 = call <vilib>:"Add State(s) to Queue__JKI_lib_State_Machine.vi"("State(s) in (\"\")"=w156) -> ("States Out"=w155:string)  [unwired: 14 in]
      }
      frame "UI: Initialize" {
        w157 = "Transconductance"
        w158 = "Conductance"
        # "Graph Labels"
        # "Initialize the User Interface, here.\n(this is called automatically, by the Macro: Init)"
        n59 = Unbundle By Name(w163) -> ("Core.Current VI Reference"=w162:refnum<vi>)
        n60 = property class="VI"(reference=w162, "Front Panel.ShowMenuBar"=TRUE ("Front Panel Window:Show Menu Bar"), "TB.Visible"=FALSE ("Front Panel Window:Show Menu Bar")) -> ()  [unwired: 1 in, 2 out]
        n61 = Bundle By Name(cluster=w163, "Paths.Path"="Path") -> (w165:T8)
        n62 = call <vilib>:"Add State(s) to Queue__JKI_lib_State_Machine.vi"("State(s) in (\"\")"=w167) -> ("States Out"=w166:string)  [unwired: 14 in]
        "String" <- w158
        "String 2" <- w157
        "String 3" <- w158
        "String 4" <- w157
      }
      frame "UI: Cursor Set" {
        # "Argument"
        # "Set and Unset Cursor Busy.\n(Usage: \"UI: Cursor Set >> Busy|Idle\")"
        n63 = case shown="\"Idle\", Default" w168 {
          tunnel: w170 -> [w175 w177]
          tunnel: [w174 w176] -> w169
          frame "Idle", Default {
            n64 = call <vilib>:"Unset Busy.vi"("error in (no error)"=w175) -> ("error out"=w174:errorcluster)  [unwired: 10 in]
          }
          frame "Busy" {
            n65 = call <vilib>:"Set Busy.vi"("error in (no error)"=w177) -> ("error out"=w176:errorcluster)  [unwired: 9 in, 1 out]
          }
        }
        n66 = call <vilib>:"Add State(s) to Queue__JKI_lib_State_Machine.vi"("State(s) in (\"\")"=w173) -> ("States Out"=w172:string)  [unwired: 14 in]
      }
      frame "UI: Front Panel State" {
        # "Argument"
        # "Set Front Panel Open or Closed\n(Usage: \"UI: Front Panel State >> Open|Close\")"
        n67 = Unbundle By Name(w180) -> ("Core.Current VI Reference"=w179:refnum<vi>)
        n68 = case shown="\"Open\", Default" w178 {
          tunnel: w182 -> [w188 w201]
          tunnel: [w190 w202] -> w181
          tunnel: w179 -> [w189 w199]
          frame "Open", Default {
            n69 = property class="VI"(reference=w189, error in=w188) -> (reference out=w186:refnum<vi>, error out=w187:errorcluster, "Front Panel.Open"=w185:bool)
            n70 = case shown="True" w185 {
              tunnel: [w193 w196] -> w190
              tunnel: w187 -> [w192 w196]
              tunnel: w186 -> [w191 _]
              frame False {
                n71 = invoke class="VI" method="FP.Open"(reference=w191, error in=w192, "Activate"=TRUE, "State"=T5."Standard") -> (error out=w193:errorcluster)  [unwired: 1 in, 4 out]
              }
              frame True {
              }
            }
          }
          frame "Close" {
            n72 = property class="VI"(reference=w199, error in=w201) -> (reference out=w198:refnum<vi>, error out=w200:errorcluster, "Front Panel.Open"=w197:bool)
            n73 = case shown="True" w197 {
              tunnel: [w203 w206] -> w202
              tunnel: w200 -> [w203 w205]
              tunnel: w198 -> [_ w204]
              frame False {
              }
              frame True {
                n74 = invoke class="VI" method="FP.Close"(reference=w204, error in=w205) -> (error out=w206:errorcluster)  [unwired: 1 in, 2 out]
              }
            }
          }
        }
        n75 = call <vilib>:"Add State(s) to Queue__JKI_lib_State_Machine.vi"("State(s) in (\"\")"=w184) -> ("States Out"=w183:string)  [unwired: 14 in]
      }
      frame "UI: Properties" {
        # "Sets offset and length of the intensity graphs."
        # "Get voltage side gate steps."
        # "Set all of the properties for the intensity graphs"
        # "This takes the B value from the  first  and last file in the folder."
        n76 = Unbundle By Name(w225) -> ("Graphs.Cond."=w220:cluster{dbl[], dbl[]}[], "Paths.Path"=w218:path, "Index/ Comments.Wavenames"=w217:string[], "B Field"=w216:i32)
        n77 = for {
          tunnel: [w230] -> w224
          tunnel: w220 -> [w229] mode=indexing
          n78 = Unbundle(w229) -> (w230:dbl[])  [unwired: 1 out]
        }
        n79 = Array Size(array=w220) -> (size(s)=w219:i32)
        n80 = call "Folder to first and last B Field.vi"("B Field"=w216, "Wavenames"=w217, "path"=w218) -> ("B Start"=w212:dbl, "B Latest"=w211:dbl)  [unwired: 7 in]
        n81 = Index Array(array=w224) -> (element #1=w221:dbl, element #2=w222:dbl)  [unwired: 2 in]
        n82 = Subtract(x=w222, y=w221) -> (x-y=w223:dbl)
        n83 = call "Scale.vi"("B_start"=w212, "B_latest"=w211, "Total_curves"=w219) -> ("output cluster"=w209:cluster{"Offset":dbl, "Multiplier":dbl})
        n84 = Unbundle(w209) -> ("Offset"=w208:dbl, "Multiplier"=w207:dbl)
        n85 = Bundle(cluster=T6 {"Offset"=0.0, "Multiplier"=0.0} ("Y Scale.Offset and Multiplier"), "Offset"=w221, "Multiplier"=w223) -> (w215:T6)
        n86 = Bundle(cluster=T6 {"Offset"=0.0, "Multiplier"=0.0} ("X Scale.Offset and Multiplier"), "Offset"=w208, "Multiplier"=w207) -> (w213:T6)
        n87 = property on="Transconductance.graph." class="IntGraph (strict)"("YScale.Ofst&Mult"=w215) -> ()  [unwired: 2 in, 2 out]
        n88 = property on="Conductance.graph." class="IntGraph (strict)"("YScale.Ofst&Mult"=w215) -> ()  [unwired: 2 in, 2 out]
        n89 = property on="Conductance. intensity" class="IntGraph (strict)"("XScale.Ofst&Mult"=w213) -> ()  [unwired: 2 in, 2 out]
        n90 = property on="Transconductance. intensity" class="IntGraph (strict)"("XScale.Ofst&Mult"=w213) -> ()  [unwired: 2 in, 2 out]
        n91 = call <vilib>:"Add State(s) to Queue__JKI_lib_State_Machine.vi"("State(s) in (\"\")"=w228) -> ("States Out"=w227:string)  [unwired: 14 in]
      }
      frame "---------- Macro ----------" {
        # "Do not put any code in this frame.\n(It is a separator no-op. You can make a copy of this frame to create a new Macro frame)"
        n92 = call <vilib>:"Add State(s) to Queue__JKI_lib_State_Machine.vi"("State(s) in (\"\")"=w234) -> ("States Out"=w233:string)  [unwired: 14 in]
      }
      frame "Macro: Initialize" {
        # "Initialization Macro\n(This is called once, when the VI starts)"
        n93 = call <vilib>:"Add State(s) to Queue__JKI_lib_State_Machine.vi"("State(s) in Front (\"\")"="Data: Initialize\nInitialize Core Data\nUI: Initialize\nUI: Front Panel State >> Open\nFile: Exist", "State(s) in (\"\")"=w239) -> ("States Out"=w238:string)  [unwired: 13 in]
      }
      frame "Macro: Conductance" {
        # "Do not put any code in this frame.\n(It is a separator no-op. You can make a copy of this frame to create a new Macro frame)"
        n94 = call <vilib>:"Add State(s) to Queue__JKI_lib_State_Machine.vi"("State(s) in Front (\"\")"="Cond: Set Index\nCond: calc\nCond: Trans\nCond: Background" ("State(s) in Front (\"\")"), "State(s) in (\"\")"=w244) -> ("States Out"=w243:string)  [unwired: 13 in]
      }
      frame "Macro: Exit" {
        # "Exit Macro\n(This is called once, when the VI exits)"
        n95 = Unbundle By Name(w252) -> ("Core.Close Panel on Exit?"=w251:bool)
        n96 = Select(t="UI: Front Panel State >> Close", s=w251, f="") -> (s? t:f=w248:string)
        n97 = call <vilib>:"Add State(s) to Queue__JKI_lib_State_Machine.vi"("State(s) in (\"\")"=w248, "State(s) at Back (\"\")"="Data: Cleanup\nExit") -> ("States Out"=w246:string)  [unwired: 13 in]
        n98 = call <vilib>:"Add State(s) to Queue__JKI_lib_State_Machine.vi"("State(s) in Front (\"\")"=w246, "State(s) in (\"\")"=w254) -> ("States Out"=w253:string)  [unwired: 13 in]
      }
      frame "---------- File ----------" {
        # "Template Separator\n(You can make a copy of, or modify, this frame)"
        n99 = call <vilib>:"Add State(s) to Queue__JKI_lib_State_Machine.vi"("State(s) in (\"\")"=w258) -> ("States Out"=w257:string)  [unwired: 14 in]
      }
      frame "File: Exist" {
        # "This state checks to ensure a file exists in order to avoid an error"
        n100 = Unbundle By Name(w267) -> ("Paths.Path"=w266:path)
        n101 = call <vilib>:"Recursive File List.vi"("error in (no error)"=w260, "Folder Path"=w266) -> ("error out"=w259:errorcluster, "Number of Files"=w265:i32)  [unwired: 5 in, 3 out]
        n102 = Equal To 0?(x=w265) -> (x = 0?=w264:bool)
        n103 = Select(t="" ("State(s) in Front (\"\")"), s=w264, f="Macro: Conductance") -> (s? t:f=w261:string)
        n104 = call <vilib>:"Add State(s) to Queue__JKI_lib_State_Machine.vi"("State(s) in Front (\"\")"=w261, "State(s) in (\"\")"=w269) -> ("States Out"=w268:string)  [unwired: 13 in]
      }
      frame "---------- Cond ----------" {
        # "Template Separator\n(You can make a copy of, or modify, this frame)"
        n105 = call <vilib>:"Add State(s) to Queue__JKI_lib_State_Machine.vi"("State(s) in (\"\")"=w273) -> ("States Out"=w272:string)  [unwired: 14 in]
      }
      frame "Cond: Set Index" {
        # "takes the values from the automatic index and converts them into the needed values for the program."
        # "Sets which index is visible and which one is not."
        # "Takes the index from the notes. If the index is not in the notes, then it will return an empty value which isnt an issue."
        # "is the index manually input or automatic?"
        # "property nodes are to show the values of the wavenames corresponding to the indices."
        n106 = Unbundle By Name(w287) -> ("Paths.Path"=w291:path)
        n107 = call "Wavenames and comments.vi"("Path"=w291) -> ("Array"=w278:string[], "Notes"=w288:string)
        n108 = call "Notes to index V2.vi"("Notes In"=w288) -> ("Comments Out"=w289:string, "output cluster"=w290:T13)  [unwired: 8 in]
        n109 = case shown="False" "Index" {
          tunnel: w278 -> [w296 w303]
          tunnel: w290 -> [_ w300]
          tunnel: ["Index." w300] -> w283
          tunnel: w289 -> [_ w304]
          tunnel: w288 -> [w299 _]
          tunnel: [w299 w304] -> w275
          frame False {
            n110 = property on="B Field" class="Ring (strict)"("Strings []"=w296) -> ()  [unwired: 2 in, 2 out]
            n111 = property on="Voltage 2" class="Ring (strict)"("Strings []"=w296) -> ()  [unwired: 2 in, 2 out]
            n112 = property on="Voltage 1" class="Ring (strict)"("Strings []"=w296) -> ()  [unwired: 2 in, 2 out]
            n113 = property on="Current" class="Ring (strict)"("Strings []"=w296) -> ()  [unwired: 2 in, 2 out]
            n114 = property on="Side Gate" class="Ring (strict)"("Strings []"=w296) -> ()  [unwired: 2 in, 2 out]
            n115 = property on="Index." class="Clust (strict)"("Visible"=TRUE) -> ()  [unwired: 2 in, 2 out]
            n116 = property on="Index" class="Clust (strict)"("Visible"=FALSE) -> ()  [unwired: 2 in, 2 out]
          }
          frame True {
            n117 = property on="Index" class="Clust (strict)"("Visible"=TRUE) -> ()  [unwired: 2 in, 2 out]
            n118 = property on="Index." class="Clust (strict)"("Visible"=FALSE) -> ()  [unwired: 2 in, 2 out]
            n119 = property on="Side Gate" class="Ring (strict)"("Strings []"=w303) -> ()  [unwired: 2 in, 2 out]
            n120 = property on="Current" class="Ring (strict)"("Strings []"=w303) -> ()  [unwired: 2 in, 2 out]
            n121 = property on="Voltage 1" class="Ring (strict)"("Strings []"=w303) -> ()  [unwired: 2 in, 2 out]
            n122 = property on="Voltage 2" class="Ring (strict)"("Strings []"=w303) -> ()  [unwired: 2 in, 2 out]
            n123 = property on="B Field" class="Ring (strict)"("Strings []"=w303) -> ()  [unwired: 2 in, 2 out]
            "Index" <- w300
          }
        }
        n124 = Unbundle By Name(w283) -> ("Side Gate"=w284:i32, "Current"=w282:i32, "Voltage 1"=w281:i32, "Voltage 2"=w280:i32, "B Field"=w277:i32, "Voltage"=w276:bool)
        n125 = Bundle By Name(cluster=T7 {"N1"=18, "N2"=19, "N3"=4, "N4"=5, "V1"=8, "V2"=10, "V3"=10, "V4"=13, "CURRENT"=12, "Vsg"=1} ("Index"), "Vsg"=w284, "CURRENT"=w282, "V1"=w281, "V2"=w280) -> (w279:T7)
        n126 = Bundle By Name(cluster=w287, "Index/ Comments.Wavenames"=w278, "Index/ Comments.Comments"=w275, "Index/ Comments.Index"=w279, "B Field"=w277, "Boolean Values.single ended?"=w276) -> (w286:T8)
        n127 = call <vilib>:"Add State(s) to Queue__JKI_lib_State_Machine.vi"("State(s) in (\"\")"=w294) -> ("States Out"=w293:string)  [unwired: 14 in]
      }
      frame "Cond: calc" {
        # "creates a 3D intensity graph"
        # "All of the heavy lifting is done by this subVI. It creates the array and fills in the blank spots where files are missing, or replaces the blank spots if files are then added."
        n128 = Unbundle By Name(w311) -> ("Paths.Path"=w310:path, "Graphs.Cond."=w308:cluster{dbl[], dbl[]}[], "Boolean Values.single ended?"=w307:bool, "Index/ Comments.Index"=w306:T7)
        n129 = call "Brain.vi"("Index"=w306, "voltage"=w307, "Conductance In"=w308, "Folder Path"=w310) -> ("Conductance Out"=w309:T3)  [unwired: 7 in]
        n130 = for {
          tunnel: w309 -> [w317] mode=indexing
          tunnel: [w316] -> w305 mode=indexing
          n131 = Unbundle(w317) -> ("Decimated Array"=w316:dbl[])  [unwired: 1 out]
        }
        n132 = Bundle By Name(cluster=w311, "Graphs.Cond."=w309, "Graphs.Cond. Intens."=w305) -> (w312:T8)
        n133 = call <vilib>:"Add State(s) to Queue__JKI_lib_State_Machine.vi"("State(s) in (\"\")"=w315) -> ("States Out"=w314:string)  [unwired: 14 in]
      }
      frame "Cond: Trans" {
        # "Takes the derivative of of each curve to calculate the transconductance."
        n134 = Unbundle By Name(w318) -> ("Graphs.Cond."=w322:cluster{dbl[], dbl[]}[])
        n135 = for {
          tunnel: [w329] -> w321 mode=indexing
          tunnel: [w328] -> w319 mode=indexing
          tunnel: w322 -> [w327] mode=indexing
          n136 = call <userlib>:"differential.vi"("Numeric"="Derivative Bin \nSize", "dy/dx vs x"=TRUE, "A vs B 2"=w327) -> ("A vs B 3"=w329:T14)  [unwired: 1 in]
          n137 = Unbundle(w329) -> ("Decimated Array"=w328:dbl[])  [unwired: 1 out]
        }
        n138 = Bundle By Name(cluster=w318, "Graphs.Trans."=w321, "Graphs.Trans. Intens."=w319) -> (w320:T8)
        n139 = call <vilib>:"Add State(s) to Queue__JKI_lib_State_Machine.vi"("State(s) in (\"\")"=w325) -> ("States Out"=w324:string)  [unwired: 14 in]
      }
      frame "Cond: Background" {
        # "This creates a background square wave that allows the end user to differentiate files that are missing from actual data."
        n140 = Unbundle By Name(w340) -> ("Graphs.Cond. Intens."=w338:dbl[][], "Graphs.Trans. Intens."=w337:dbl[][])
        n141 = property on="Conductance.." class="IntGraph (strict)"() -> ("ZScale.Maximum"=w334:dbl, "YScale.Maximum"=w333:dbl)  [unwired: 2 in, 2 out]
        n142 = property on="Transconductance.." class="IntGraph (strict)"() -> ("ZScale.Maximum"=w332:dbl, "YScale.Maximum"=w331:dbl)  [unwired: 2 in, 2 out]
        n143 = call "pattern maker.vi"("intensity graph in"=w338, "Z Scale.Range:Maximum"=w334, "Y Scale.Range:Maximum"=w333) -> ("Intensity graph out"=w336:dbl[][])  [unwired: 6 in]
        n144 = call "pattern maker.vi"("intensity graph in"=w337, "Z Scale.Range:Maximum"=w332, "Y Scale.Range:Maximum"=w331) -> ("Intensity graph out"=w335:dbl[][])  [unwired: 6 in]
        n145 = Bundle By Name(cluster=w340, "Graphs.Cond. Intens. bg"=w336, "Graphs.Trans. Intens. bg"=w335) -> (w339:T8)
        n146 = call <vilib>:"Add State(s) to Queue__JKI_lib_State_Machine.vi"("State(s) in (\"\")"=w343) -> ("States Out"=w342:string)  [unwired: 14 in]
      }
      frame "---------- Copy Me ----------" {
        # "Template Separator\n(You can make a copy of, or modify, this frame)"
        n147 = call <vilib>:"Add State(s) to Queue__JKI_lib_State_Machine.vi"("State(s) in (\"\")"=w347) -> ("States Out"=w346:string)  [unwired: 14 in]
      }
      frame "Copy Me" {
        # "Your code here.\n(You can make a copy of, or modify, this frame)"
        n148 = call <vilib>:"Add State(s) to Queue__JKI_lib_State_Machine.vi"("State(s) in (\"\")"=w351) -> ("States Out"=w350:string)  [unwired: 14 in]
      }
    }
  }
